vi "探头窗口-6-网络版.vi"() -> ()   [LabVIEW 2017]
panel:
  in  "外部停止命令？":bool=TRUE
  out "引用-监测模式？":refnum<vi>
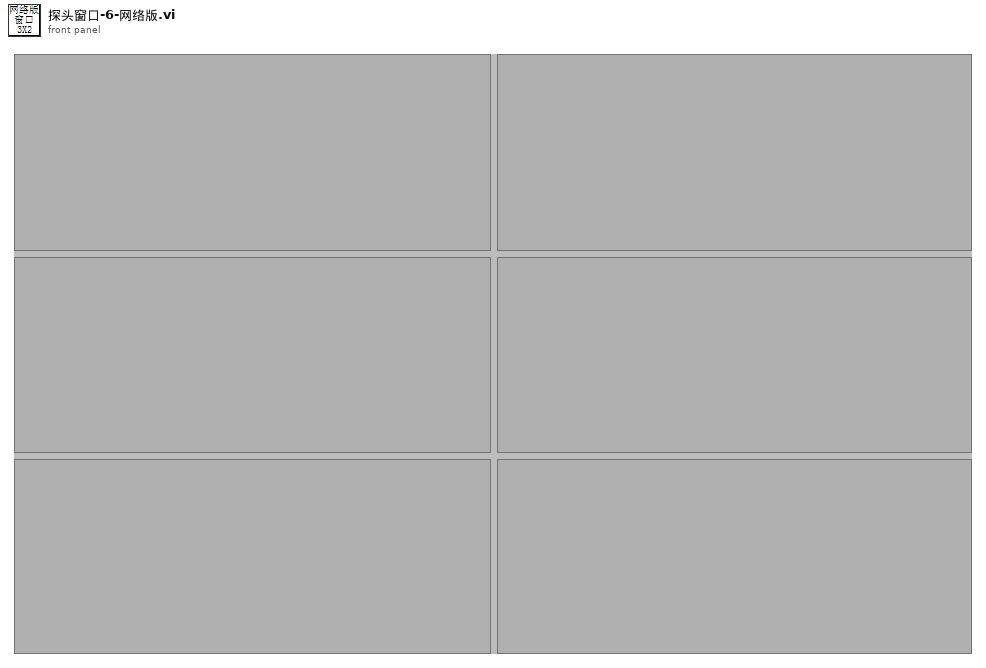
[diagram p1: front panel]
types:
  T1 = typedef "探头属性.ctl" = cluster{"探头地址与信息":T2, "测量值":T5, "限值":T6, "探头状态":T7, "累积记录":T8, "报警方式":T9}
  T2 = typedef "探测器信息.ctl" = cluster{"网络地址":string, "名称":string, "备注":string, "累积剂量":dbl, "累积限值":dbl, "硬件剂量率限值":T3, "剂量率限值1":dbl, "剂量率限值2":dbl, "报警方式":T4}
  T3 = typedef "探头剂量率限值选择.ctl" = enum16{"一级限值", "二级限值"}
  T4 = typedef "报警方式选择.ctl" = enum16{"常报警", "自动静音", "手动静音"}
  T5 = typedef "测量值.ctl" = cluster{"时间":timestamp, "数值":dbl}
  T6 = typedef "剂量率限值.ctl" = cluster{"限值1":dbl, "限值2":dbl, "探头限值":T3}
  T7 = typedef "探头状态.ctl" = enum16{"正常", "离线", "禁用", "一级报警", "二级报警", "累积报警"}
  T8 = typedef "单条累积记录.ctl" = cluster{"起始时间":timestamp, "结束时间":timestamp, "累积剂量":dbl}
  T9 = typedef "报警方式.ctl" = cluster{"报警方式":T4, "延迟计时":u16, "报警中？":bool}
  T10 = typedef "eventvkey.ctl" = enum16{"ASCII", "Enter", "Return", "Shift", "Ctrl", "Alt", "Cmd", "Opt", "Caps", "NumLock", "Clear", "Break", "Up", "Down", "Left", "Right", "Insert", "Delete", "Home", "End", "PageUp", "PageDown", "Escape", "Help", "Pause", "ScrollLock", "F1", "F2", "F3", "F4", "F5", "F6", "F7", "F8", "F9", "F10", "F11", "F12", "F13", "F14", "F15", "F16", "F17", "F18", "F19", "F20", "F21", "F22", "F23", "F24", "Play", "VolumeUp", "VolumeDown", "Mute", "Two Byte Char"}
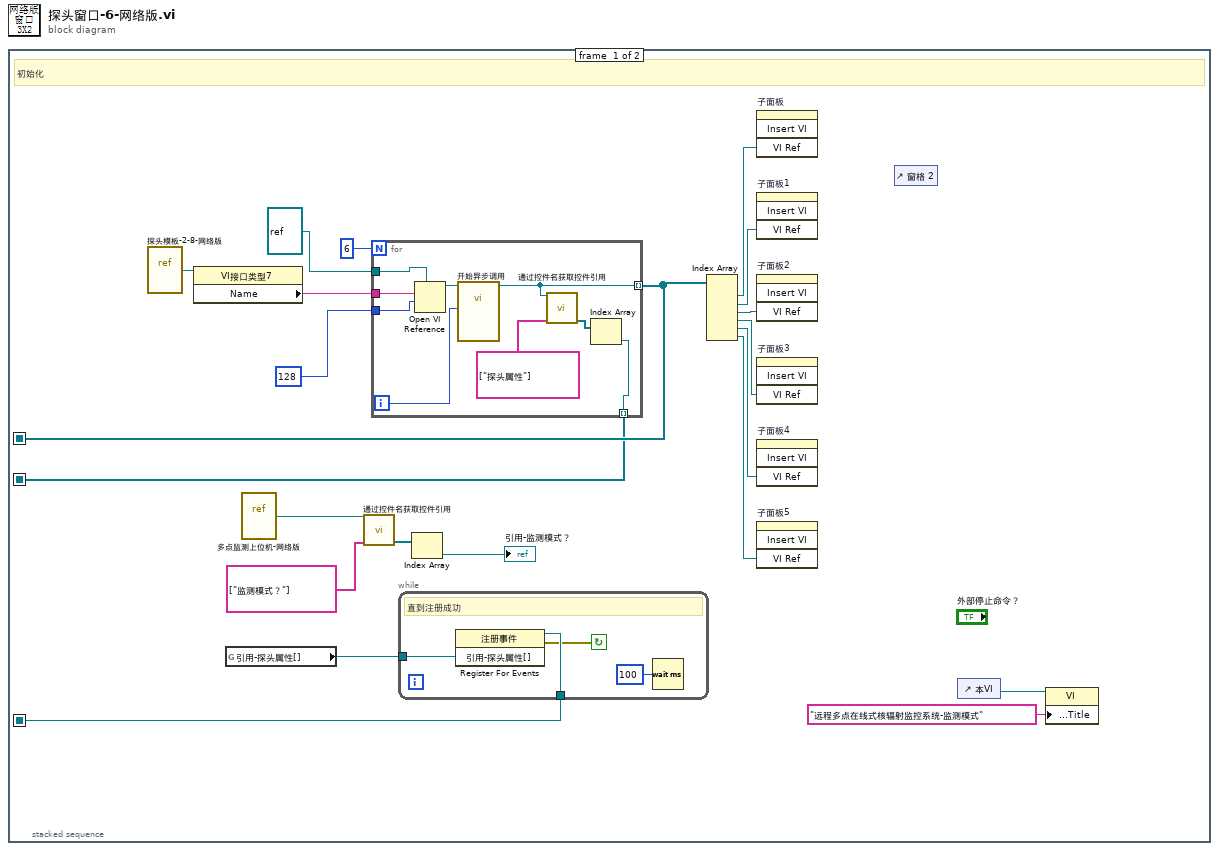
[diagram p0: block diagram]
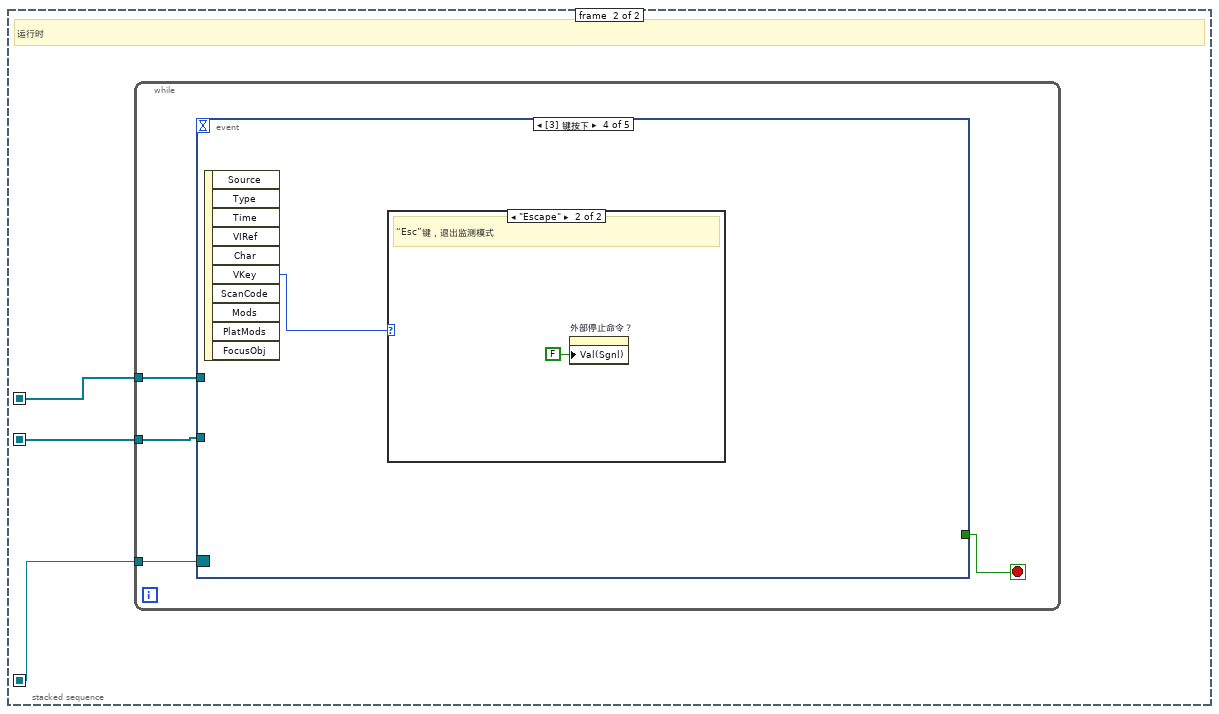
[diagram p2: hidden frame]
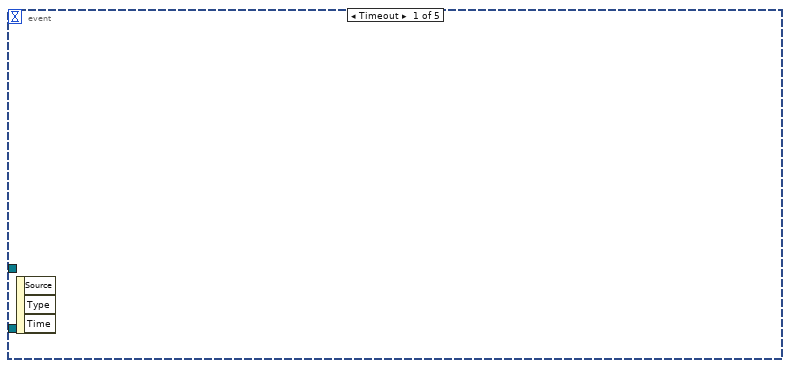
[diagram p3: hidden frame]
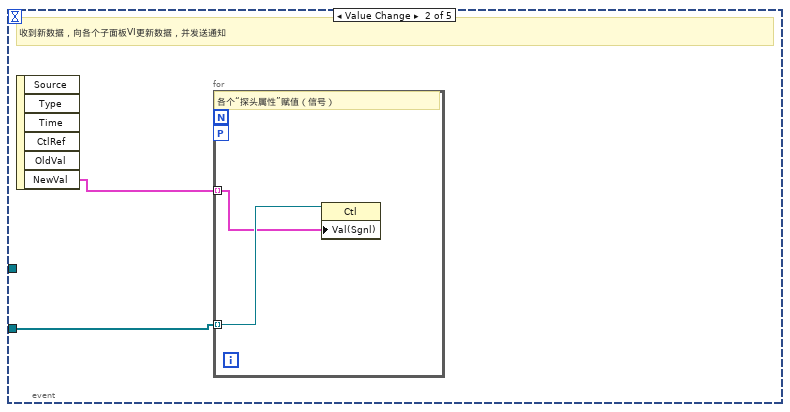
[diagram p4: hidden frame]
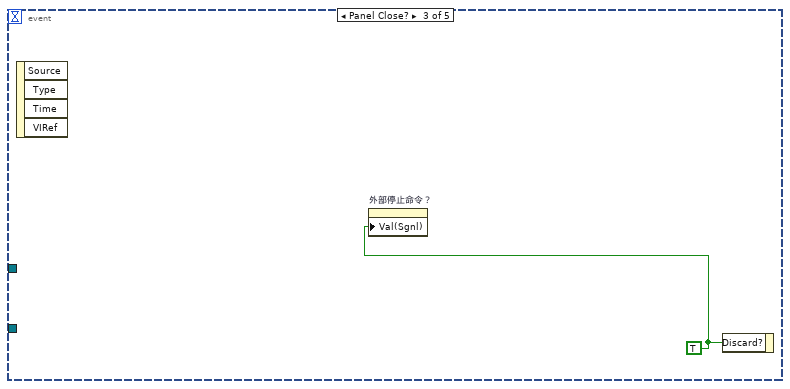
[diagram p5: hidden frame]
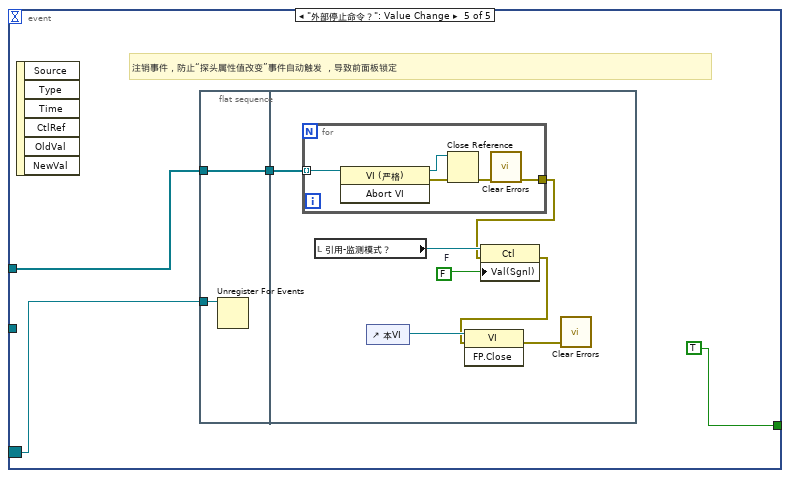
[diagram p7: hidden frame]
diagram:
  n1 = stacked-sequence {
    seq-local: [w17 _] -> [_ w37]
    seq-local: [w9 _] -> [_ w36]
    seq-local: [w1 _] -> [_ w35]
    frame #0 {
      # "初始化"
      n2 = vi-ref "探头模板-2-8-网络版.vi"() -> (w21:refnum<vi>)
      n3 = property class="VI接口类型7"(reference=w21) -> ("Name"=w20:string)  [unwired: 1 in, 2 out]
      n4 = global read "全局变量-35点监测.vi" "引用-探头属性[]"() -> (w2:refnum<vi>)
      n5 = vi-ref "多点监测上位机-网络版.vi"() -> (w5:refnum<vi>)
      n6 = call "通过控件名获取控件引用.vi"("控件名数组"=string[] ["监测模式？"], "VI引用"=w5) -> ("控件引用输出"=w7:refnum<vi>[])  [unwired: 7 in, 2 out]
      n7 = for {
        N: 6 -> [_]
        tunnel: w20 -> [w34]
        tunnel: 128 ("选项") -> [w33]
        tunnel: refnum<vi> refnum ("类型说明符VI引用句柄（仅用于类型）") -> [w32]
        tunnel: [w27] -> w17 mode=indexing
        tunnel: [w28] -> w9 mode=indexing
        i -> [w26]
        n8 = Open VI Reference(type specifier VI Refnum (for type only)=w32, vi path=w34, options=w33) -> (vi reference=w29:refnum<vi>)  [unwired: 3 in, 1 out]
        n9 = call-by-ref "开始异步调用"(reference=w29, "探头序号"=w26) -> (reference out=w27:refnum<vi>)  [unwired: 12 in, 1 out]
        n10 = call "通过控件名获取控件引用.vi"("控件名数组"=string[] ["探头属性"], "VI引用"=w27) -> ("控件引用输出"=w31:refnum<vi>[])  [unwired: 7 in, 2 out]
        n11 = Index Array(array=w31) -> (element=w28:refnum<vi>)  [unwired: 1 in]
      }
      n12 = while {
        tunnel: w2 -> [w25]
        tunnel: [w24] -> w1
        stop <- w23 continue-if-true
        # "直到注册成功"
        n13 = register-events(w25) -> (reference out=w24:refnum<event-registration>, error out=w23:errorcluster)  [unwired: 2 in]
        n14 = Wait (ms)(milliseconds to wait=u32 100 ("等待时间（毫秒）")) -> ()  [unwired: 1 out]
      }
      n15 = Index Array(array=w7) -> (element=→"引用-监测模式？":refnum<vi>)  [unwired: 1 in]
      n16 = Index Array(array=w17) -> (element #1=w15:refnum<vi>, element #2=w14:refnum<vi>, element #3=w13:refnum<vi>, element #4=w12:refnum<vi>, element #5=w10:refnum<vi>, element #6=w11:refnum<vi>)  [unwired: 6 in]
      n17 = invoke on="子面板" class="子面板" method="Insert VI"("VI Ref"=w15) -> ()  [unwired: 3 in, 4 out]
      n18 = invoke on="子面板1" class="SubPnl" method="Insert VI"("VI Ref"=w14) -> ()  [unwired: 3 in, 4 out]
      n19 = invoke on="子面板2" class="SubPnl" method="Insert VI"("VI Ref"=w13) -> ()  [unwired: 3 in, 4 out]
      n20 = invoke on="子面板3" class="SubPnl" method="Insert VI"("VI Ref"=w12) -> ()  [unwired: 3 in, 4 out]
      n21 = invoke on="子面板4" class="SubPnl" method="Insert VI"("VI Ref"=w10) -> ()  [unwired: 3 in, 4 out]
      n22 = invoke on="子面板5" class="SubPnl" method="Insert VI"("VI Ref"=w11) -> ()  [unwired: 3 in, 4 out]
      n23 = control-ref of="窗格 2"() -> ()  [unwired: 1 out]
      n24 = control-ref of="本VI"() -> (w4:refnum<vi>)
      n25 = property class="VI"(reference=w4, "Front Panel.Title"="远程多点在线式核辐射监控系统-监测模式" ("前面板窗口:标题")) -> ()  [unwired: 1 in, 2 out]
    }
    frame #1 {
      # "运行时"
      n26 = while {
        tunnel: w37 -> [w40]
        tunnel: w36 -> [w39]
        tunnel: w35 -> [w38]
        stop <- w41 stop-if-true
        n27 = event shown="[3] 键按下" {
          selector: w38 -> [_ _ _ _ w49]
          dyn-events: _ -> [_ _ _ _ _]
          timeout: _ -> [_ _ _ _ _]
          tunnel: [_ _ _ _ TRUE ("放弃？")] -> w41
          tunnel: w40 -> [_ _ _ _ w51]
          tunnel: w39 -> [_ w42 _ _ _]
          event Timeout {
            n28 = event-data() -> ()  [unwired: 1 in, 3 out]
          }
          event Value Change {
            # "收到新数据，向各个子面板VI更新数据，并发送通知"
            n29 = event-data() -> ("NewVal"=w43:T1[])  [unwired: 1 in, 5 out]
            n30 = for {
              workers-P: _ -> [_]
              tunnel: w42 -> [w45] mode=indexing
              tunnel: w43 -> [w44] mode=indexing
              # "各个“探头属性”赋值（信号）"
              n31 = property class="Ctl"(reference=w45, "Val(Sgnl)"=w44) -> ()  [unwired: 1 in, 2 out]
            }
          }
          event Panel Close? {
            w46 = TRUE ("放弃？")
            n32 = event-data() -> ()  [unwired: 1 in, 4 out]
            n33 = property on="外部停止命令？" class="Bool (严格)"("Val(Sgnl)"=w46) -> ()  [unwired: 2 in, 2 out]
            n34 = event-data("Discard?"=w46) -> ()  [unwired: 1 in, 1 out]
          }
          event Key Down {
            n35 = event-data() -> ("VKey"=w47:T10)  [unwired: 1 in, 9 out]
            n36 = case shown="\"Escape\"" w47 {
              frame "ASCII", Default {
              }
              frame "Escape" {
                # "“Esc”键，退出监测模式"
                n37 = property on="外部停止命令？" class="Bool (严格)"("Val(Sgnl)"=FALSE ("值(信号)")) -> ()  [unwired: 2 in, 2 out]
              }
            }
          }
          event "外部停止命令？": Value Change {
            # "注销事件，防止“探头属性值改变”事件自动触发 ，导致前面板锁定"
            n38 = event-data() -> ()  [unwired: 1 in, 6 out]
            n39 = flat-sequence {
              tunnel: w51 -> [w54]
              tunnel: [w54] -> w50
              tunnel: w49 -> [w53]
              tunnel: w50 -> [w61]
              frame #0 {
                n40 = Unregister For Events(event registration refnum=w53) -> ()  [unwired: 1 in, 1 out]
              }
              frame #1 {
                w60 = FALSE  # F
                n41 = for {
                  tunnel: w61 -> [w66] mode=indexing
                  tunnel: [w62] -> w57
                  n42 = invoke class="VI (严格)" method="Abort VI"(reference=w66) -> (reference out=w64:refnum<vi>, error out=w65:errorcluster)  [unwired: 2 in, 1 out]
                  n43 = Close Reference(reference=w64, error in (no error)=w65) -> (error out=w63:errorcluster)
                  n44 = call <vilib>:"Clear Errors.vi"("error in (no error)"=w63) -> ("error out"=w62:errorcluster)  [unwired: 5 in, 1 out]
                }
                n45 = local read "引用-监测模式？"() -> (w59:refnum<vi>)
                n46 = control-ref of="本VI"() -> (w58:refnum<vi>)
                n47 = property class="Ctl"(reference=w59, error in=w57, "Val(Sgnl)"=w60) -> (error out=w56:errorcluster)  [unwired: 1 out]
                n48 = invoke class="VI" method="FP.Close"(reference=w58, error in=w56) -> (error out=w55:errorcluster)  [unwired: 1 in, 2 out]
                n49 = call <vilib>:"Clear Errors.vi"("error in (no error)"=w55) -> ()  [unwired: 5 in, 2 out]
              }
            }
          }
        }
      }
    }
  }
